vi "pp2_log_trialMemo.vi"(10 "queue in":refnum<queue>) -> (2 "queue out":refnum<queue>)   [LabVIEW 2013]
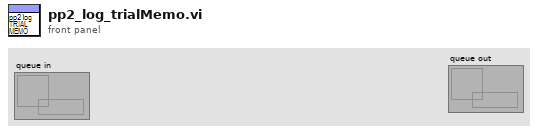
[diagram p1: front panel]
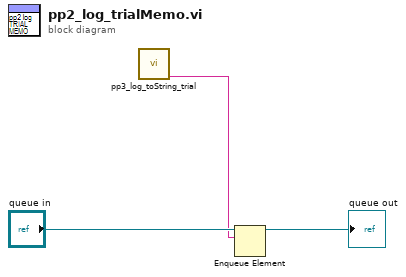
[diagram p0: block diagram]
diagram:
  n1 = call "pp3_log_toString_trial.vi"() -> ("TRIALMEMO String"=w1:string)  [unwired: 10 in, 1 out]
  n2 = Enqueue Element(queue="queue in", element=w1) -> (queue out=→"queue out":refnum<queue>)  [unwired: 2 in, 2 out]
